vi "Configure IQ vs Slot Measurement List Range.vi"(6 "Stop Index (19)":i32=19, 7 "Start Index (0)":i32 format="%.0g", 8 "error in (no error)":errorcluster, 9 "State (Off)":bool, 10 "Instance (1)":i32=1 format="%.0g", 11 "VISA resource name":refnum<visa-resource-name>) -> (0 "error out":errorcluster, 3 "VISA resource name out":refnum<visa-resource-name>)   [LabVIEW 2015, in "Rohde&Schwarz CMXP GPRF.lvlib"]
doc: "Configures state, start and stop index of IQ vs Slot measurement list mode.\n\nAttributes:\nRSCMXPGPRF_ATTR_IQ_VS_SLOT_MEASUREMENT_LIST_MODE_STATE\nRSCMXPGPRF_ATTR_IQ_VS_SLOT_MEASUREMENT_LIST_START\nRSCMXPGPRF_ATTR_IQ_VS_SLOT_MEASUREMENT_LIST_STOP\n\nRemote-control commands:\nCONFigure:GPRF:MEAS<i>:IQVSlot:LIST\nCONFigure:GPRF:MEAS<i>:IQVSlot:LIST:STARt\nCONFigure:GPRF:MEAS<i>:IQVSlot:LIST:STOP"
uses:
  <instrlib>/Rohde&Schwarz CMXP GPRF/Rohde&Schwarz CMXP GPRF.lvlib
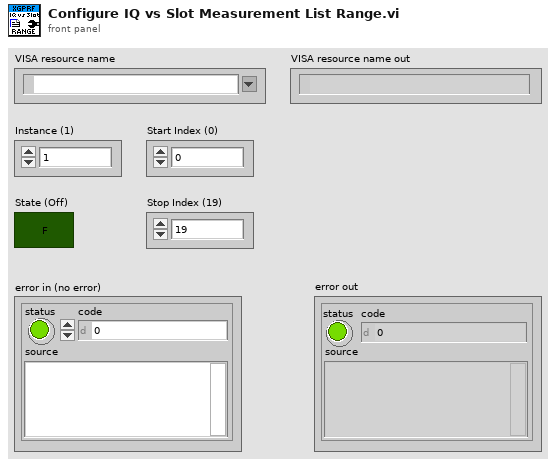
[diagram p1: front panel]
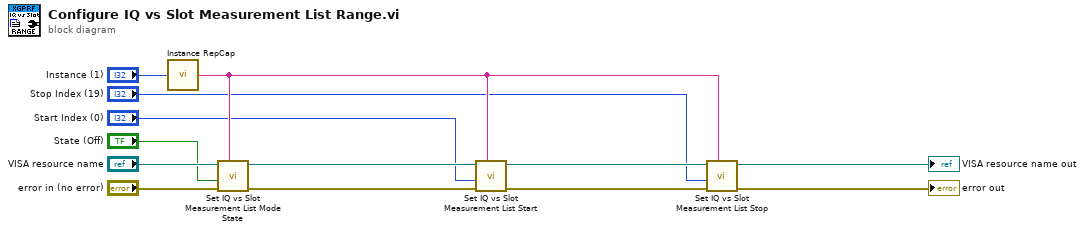
[diagram p0: block diagram]
diagram:
  n1 = call <instrlib>:"Instance RepCap.vi"("instance  in"="Instance (1)") -> ("instance out"=w13:string)
  n2 = call "Set IQ vs Slot Measurement List Mode State"("Repeated Capabilities"=w13, "error in (no error)"="error in (no error)", "IQ vs Slot Measurement List Mode State (OFF)"="State (Off)", "instrument handle"="VISA resource name") -> ("error out"=w12:errorcluster, "instrument handle out"=w11:refnum<visa-resource-name>)  [unwired: 6 in]
  n3 = call "Set IQ vs Slot Measurement List Start"("Repeated Capabilities"=w13, "error in (no error)"=w12, "IQ vs Slot Measurement List Start (0)"="Start Index (0)", "instrument handle"=w11) -> ("error out"=w9:errorcluster, "instrument handle out"=w10:refnum<visa-resource-name>)  [unwired: 6 in]
  n4 = call "Set IQ vs Slot Measurement List Stop"("Repeated Capabilities"=w13, "error in (no error)"=w9, "IQ vs Slot Measurement List Stop (0)"="Stop Index (19)", "instrument handle"=w10) -> ("error out"=→"error out":errorcluster, "instrument handle out"=→"VISA resource name out":refnum<visa-resource-name>)  [unwired: 6 in]
